vi "Get Control Panel VI Path.vi"(8 "error in (no error)":errorcluster, 11 "Neocera LTC-21 in":refnum<class "Neocera LTC-21.lvclass">) -> (0 "error out":errorcluster, 2 "Front Panel VI path":path, 3 "Neocera LTC-21 out":refnum<class "Neocera LTC-21.lvclass">)   [LabVIEW 2015, in "Neocera LTC-21.lvclass"]
uses:
  Neocera LTC-21.lvclass
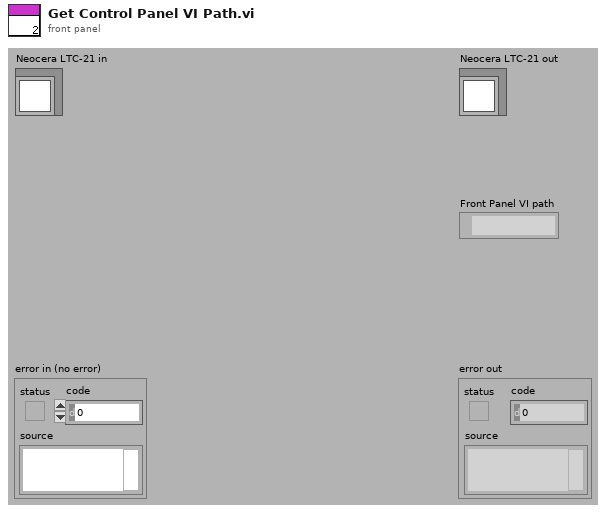
[diagram p1: front panel]
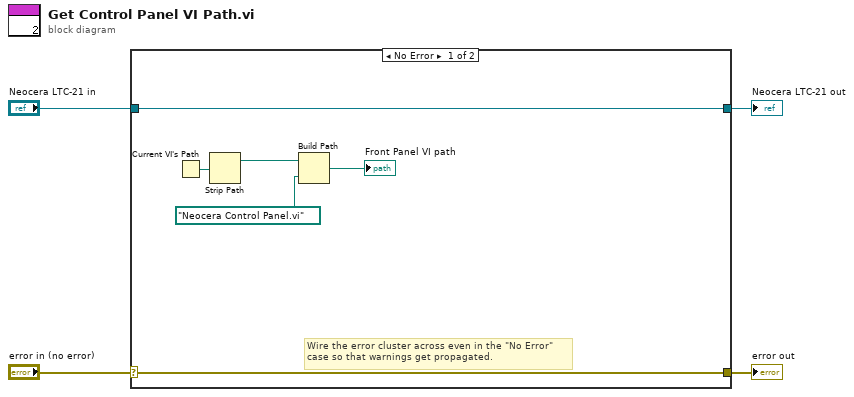
[diagram p0: block diagram]
diagram:
  n1 = case shown="No Error" "error in (no error)" {
    selector: "error in (no error)" -> [w9 w12]
    tunnel: [w9 w12] -> w3
    tunnel: [w10 w11] -> w1
    tunnel: "Neocera LTC-21 in" -> [w10 w11]
    frame No Error {
      # "Wire the error cluster across even in the \"No Error\"\ncase so that warnings get propagated."
      n2 = Current VI's Path() -> (path=w7:path)
      n3 = Strip Path(path=w7) -> (stripped path=w6:path)  [unwired: 1 out]
      n4 = Build Path(base path=w6, name or relative path=path "Neocera Control Panel.vi") -> (appended path=→"Front Panel VI path":path)
    }
    frame Error {
    }
  }
  "error out" <- w3
  "Neocera LTC-21 out" <- w1
